vi "6.4.1.vi"() -> ()   [LabVIEW 2018]
panel:
  in  "읽어올 경로":path
  out "웨이브폼 차트":dbl[](graph)
  in  "저장경로":path
  out "데이터":dbl[](array[numeric])
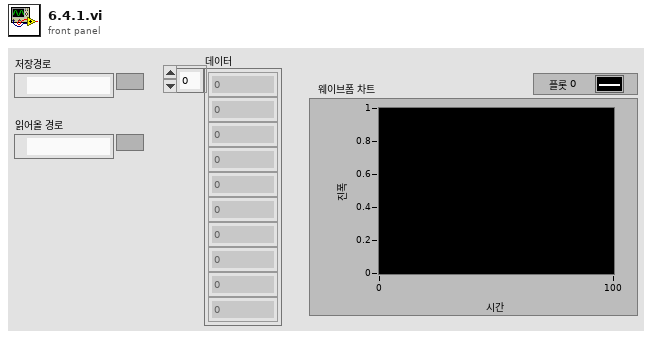
[diagram p1: front panel]
types:
  T1 = enum16{"open", "replace", "create", "open or create", "replace or create", "replace or create with confirmation"}
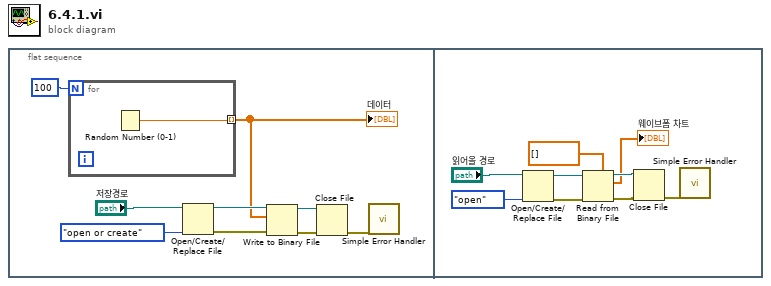
[diagram p0: block diagram]
diagram:
  n1 = flat-sequence {
    frame #0 {
      n2 = for {
        N: 100 -> [_]
        tunnel: [w10] -> w1 mode=indexing
        n3 = Random Number (0-1)() -> (number: 0 to 1=w10:dbl)
      }
      "데이터" <- w1
      n4 = Open/Create/Replace File(file path (use dialog)="저장경로", operation (0:open)=T1."open or create" ("동작(0:open)")) -> (refnum out=w3:refnum<file>, error out=w5:errorcluster)  [unwired: 4 in, 1 out]
      n5 = Write to Binary File(file (use dialog)=w3, data=w1, error in=w5) -> (refnum out=w2:refnum<file>, error out=w4:errorcluster)  [unwired: 3 in, 1 out]
      n6 = Close File(refnum=w2, error in=w4) -> (error out=w6:errorcluster)  [unwired: 1 out]
      n7 = call <vilib>:"Simple Error Handler.vi"("error in (no error)"=w6) -> ()  [unwired: 4 in, 5 out]
    }
    frame #1 {
      n8 = Open/Create/Replace File(file path (use dialog)="읽어올 경로", operation (0:open)=T1."open" ("동작(0:open)")) -> (refnum out=w14:refnum<file>, error out=w15:errorcluster)  [unwired: 4 in, 1 out]
      n9 = Read from Binary File(5:dbl[] [], 8:w15, 11:w14) -> (0:w16:errorcluster, 2:→"웨이브폼 차트":dbl[], 3:w13:refnum<file>)  [unwired: 3 in, 1 out]
      n10 = Close File(refnum=w13, error in=w16) -> (error out=w17:errorcluster)  [unwired: 1 out]
      n11 = call <vilib>:"Simple Error Handler.vi"("error in (no error)"=w17) -> ()  [unwired: 4 in, 5 out]
    }
  }
